vi "The Most Near Color.vi"(2 "Temperature Limit":dbl, 3 "Min Temperature":dbl, 4 "Max Temperature":dbl) -> (0 "Closest Temperature":dbl, 1 "Closest Color":u32)   [LabVIEW 2016]
uses:
  Global Flir-Ax8.vi
  <vilib>/imath/engines/lvmath2/RunTimeEngine/BuiltInFunctions/rotate90/NIMS_rotate90.vi
  <instcachedir>/0/NIMS_rotate90_7DC1660D109944E092D2EB6E3185A1B6.lvgen/NIMS_rotate90_7DC1660D109944E092D2EB6E3185A1B6_004.vi
  <vilib>/imath/engines/lvmath2/RunTimeEngine/BuiltInFunctions/mirrorh/NIMS_mirrorh(GM).vi
  <instcachedir>/0/NIMS_mirrorh(GM)_A650AD0D730A4A8EBE251B4C5C7CA115.lvgen/NIMS_mirrorh(GM)_A650AD0D730A4A8EBE251B4C5C7CA115_004.vi
  <vilib>/imath/engines/lvmath2/RunTimeEngine/BuiltInFunctions/length/NIMS_length(GM).vi
  <instcachedir>/0/NIMS_length(GM)_47CEC356FCE0482D9BA47DC61C99F2C7.lvgen/NIMS_length(GM)_47CEC356FCE0482D9BA47DC61C99F2C7_006.vi
  <vilib>/imath/engines/lvmath2/RunTimeEngine/IndexReplace/NIMS V(S)=S.vi
  <instcachedir>/0/NIMS V(S)=S_57E16554CB8B4B90AAB163894F717546.lvgen/NIMS V(S)=S_57E16554CB8B4B90AAB163894F717546_000.vi
  <vilib>/imathl/engines/lvmath/Functions/Error Handling/Create Error.vi
  <vilib>/imath/engines/lvmath2/RunTimeEngine/RangeToken/NIMS_Range_R2 - Integer.vi
  <instcachedir>/0/NIMS_Range_R2 - Integer_89B873E74E6E489885E44F751DD9C6BF.lvgen/NIMS_Range_R2 - Integer_89B873E74E6E489885E44F751DD9C6BF_000.vi
  <vilib>/imath/engines/lvmath2/RunTimeEngine/CommandStatement/MC_CommandStatement_break.vi
  <vilib>/imath/engines/lvmath2/RunTimeEngine/BuiltInFunctions/mirrorh/NIMS_mirrorh(GRowV).vi
  <instcachedir>/0/NIMS_mirrorh(GRowV)_B6A8CC4EAFBA4F9A82A59460D67BDFF0.lvgen/NIMS_mirrorh(GRowV)_B6A8CC4EAFBA4F9A82A59460D67BDFF0_000.vi
  <vilib>/imath/engines/lvmath2/RunTimeEngine/IndexRead/NIMS V($).vi
  <instcachedir>/0/NIMS V($)_C593F32C7F6B43C7B1793952E292524F.lvgen/NIMS V($)_C593F32C7F6B43C7B1793952E292524F_001.vi
  <vilib>/imath/engines/lvmath2/RunTimeEngine/NodeEndStatement/NIMS_NodeEndStatement_Output.vi
  <instcachedir>/0/NIMS_NodeEndStatement_Output_53EC0D466D134D7ABD903AC30B43404B.lvgen/NIMS_NodeEndStatement_Output_53EC0D466D134D7ABD903AC30B43404B_005.vi
  <vilib>/imath/engines/lvmath2/RunTimeEngine/ErrorHandling/NIMS_Finalize Error.vi
panel:
  out "Color Palette":u32[][](array[numeric])
  out "Closest Index":i32
  out "Temperature Vector":dbl[](array[numeric])
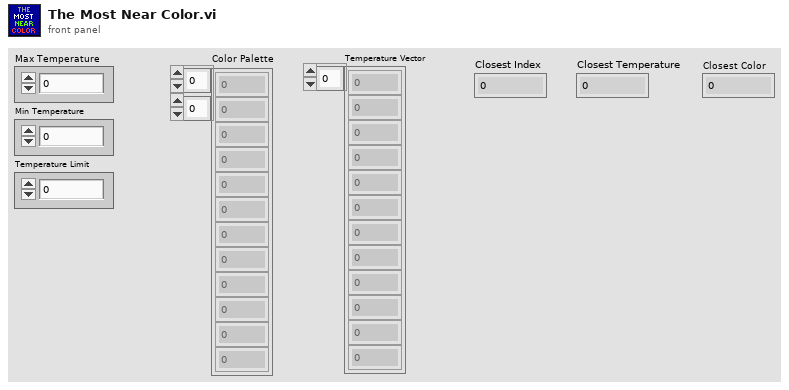
[diagram p1: front panel]
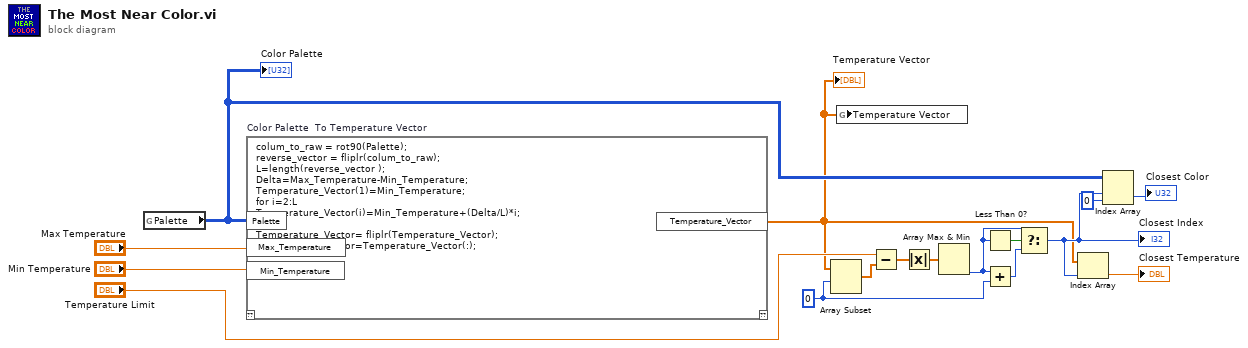
[diagram p0: block diagram]
diagram:
  w4 = 0 ("start index (0)")
  n1 = global read "Global Flir-Ax8.vi" "Palette"() -> (w3:u32[][])
  "Color Palette" <- w3
  n2 = mathscript code="colum_to_raw = rot90(Palette);\nreverse_vector = fliplr(colum_to_raw);\nL=length(reverse_vector );\nDelta=Max_Temperature-Min_Temperature;\nTemperature_Vector(1)=Min_Temperature;\nfor i=2:L\nTemperature_Vector(i)=Min_Temperature+(Delta/L)*i;\nend\nTemperature_Vector= fliplr(Temperature_Vector);\nTemperature_Vector=Temperature_Vector(:);" "Color Palette  To Temperature Vector"("Palette"=w3, "Max_Temperature"="Max Temperature", "Min_Temperature"="Min Temperature") -> ("Temperature_Vector"=w1:dbl[])  [unwired: 1 in, 1 out]
  "Temperature Vector" <- w1
  n3 = Array Subset(array=w1, index=w4) -> (w8:dbl[])  [unwired: 1 in]
  n4 = global write "Global Flir-Ax8.vi" "Temperature Vector"(w1) -> ()
  n5 = Subtract(x="Temperature Limit", y=w8) -> (x-y=w14:dbl[])
  n6 = Absolute Value(x=w14) -> (abs(x)=w12:dbl[])
  n7 = Array Max & Min(array=w12) -> (min index (indices)=w10:i32)  [unwired: 3 out]
  n8 = Less Than 0?(x=w10) -> (x < 0?=w11:bool)
  n9 = Add(x=w10, y=w4) -> (x+y=w9:i32)
  n10 = Select(t=w10, s=w11, f=w9) -> (s? t:f=w7:i32)
  "Closest Index" <- w7
  n11 = Index Array(array=w1, index=w7) -> (element=→"Closest Temperature":dbl)
  n12 = Index Array(array=w3, index (row)=w7, index (col)=0 ("disabled index (col)")) -> (element=→"Closest Color":u32)
